vi "DDC (Four Channels).vi"(0 "data in":T1[](array[typedef]), 1 "reset":bool, 5 "start trigger":bool, 9 "enable":bool[](array[boolean]), 11 "ddc parameters":T2[](array[typedef]) {"frequency shift" format="%#.48g"}) -> (4 "data out":u32[](array[numeric]), 6 "number of overflows":u64[](array[numeric]), 10 "output valid":bool, 14 "dsp reset done":bool)   [LabVIEW 2016]
doc: "Digital downconverter (DDC). Implemented with FPGA-based DSP.\n\n<B>Input Parameters</B>\n\n<B>data in</B> is the I and Q data to be downconverted along with overflow information.\n\n<B>start trigger</B> triggers the Rx signal chain if an Rx stream is enabled.\n\n<B>enable</B> specifies which streams are enabled.\n\n<B>ddc parameters</B> are the downconversion parameters utilized by the DSP chain.\n\n<B>reset</B> the DSP downconversion signal chain.\n\n<B>Output Parameters</B>\n\n<B>dsp reset done</B> indicates that the DSP downconversion signal chain completed reset.\n\n<B>data out</B> is the downconverted data.\n\n<B>number of overflows</B> is the number of times the DSP chain overflowed on fixed point conversion of 'data in'.\n\n<B>output valid</B> specifies when 'data out' is valid."
uses:
  <instrlib>/_niInstr/DSP/v1/Shared/Public/IQ Data.ctl
  <instrlib>/_niInstr/DSP/v1/Shared/niInstr DSP v1 Shared.lvlib
  <instrlib>/_niInstr/DSP/v1/Shared/Public/IQ Impairments.ctl
  DDC Parameters.ctl
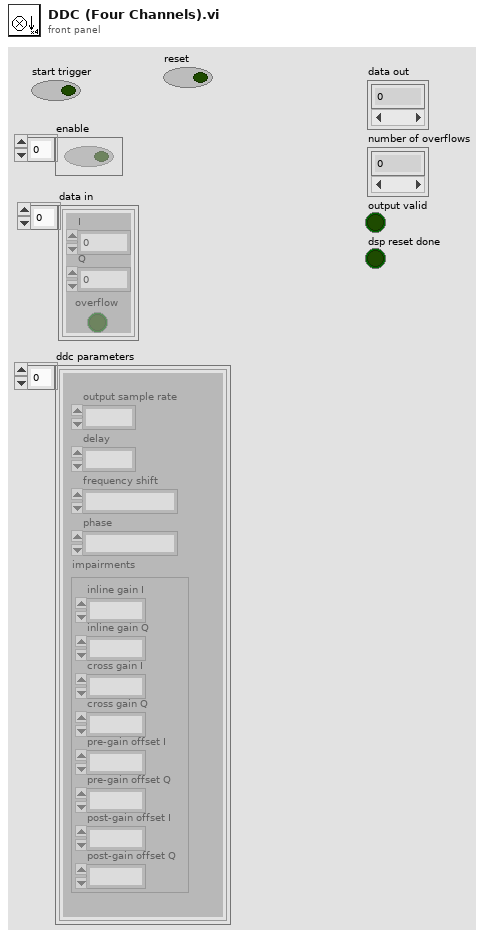
[diagram p1: front panel]
types:
  T1 = typedef "niInstr DSP v1 Shared.lvlib/IQ Data.ctl" = cluster{"I":fxp<+/-,18,1>, "Q":fxp<+/-,18,1>, "overflow":bool}
  T2 = typedef "DDC Parameters.ctl" = cluster{"output sample rate":fxp<+,48,1>, "delay":fxp<+/-,16,0>, "frequency shift":fxp<+/-,48,0>, "impairments":T3, "phase":fxp<+/-,21,0>}
  T3 = typedef "niInstr DSP v1 Shared.lvlib/IQ Impairments.ctl" = cluster{"inline gain I":fxp<+/-,18,1>, "inline gain Q":fxp<+/-,18,1>, "cross gain I":fxp<+/-,18,1>, "cross gain Q":fxp<+/-,18,1>, "pre-gain offset I":fxp<+/-,18,1>, "pre-gain offset Q":fxp<+/-,18,1>, "post-gain offset I":fxp<+/-,18,1>, "post-gain offset Q":fxp<+/-,18,1>}
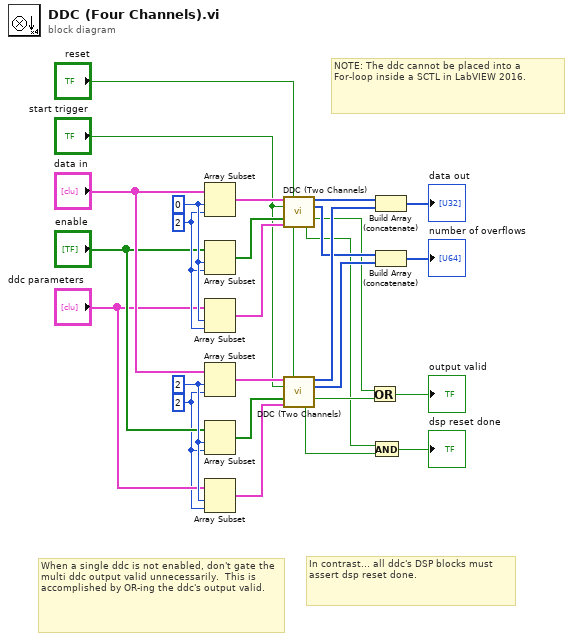
[diagram p0: block diagram]
diagram:
  w15 = 2 ("length")
  w20 = 2 ("index")
  w22 = 2 ("length")
  w23 = 0 ("index")
  # "NOTE: The ddc cannot be placed into a For-loop inside a SCTL in LabVIEW 2016."
  # "When a single ddc is not enabled, don't gate the multi ddc output valid unnecessarily.  This is accomplished by OR-ing the ddc's output valid."
  # "In contrast... all ddc's DSP blocks must assert dsp reset done."
  n1 = Array Subset(array="data in", index=w23, length=w22) -> (w25:T1[])
  n2 = Array Subset(array="enable", index=w23, length=w22) -> (w24:bool[])
  n3 = Array Subset(array="ddc parameters", index=w23, length=w22) -> (w21:T2[])
  n4 = Array Subset(array="data in", index=w20, length=w15) -> (w16:T1[])
  n5 = Array Subset(array="enable", index=w20, length=w15) -> (w13:bool[])
  n6 = Array Subset(array="ddc parameters", index=w20, length=w15) -> (w14:T2[])
  n7 = call "DDC (Two Channels).vi"("data in"=w25, "reset"="reset", "start trigger"="start trigger", "enable"=w24, "ddc parameters"=w21) -> ("data out"=w10:u32[], "number of overflows"=w6:u64[], "output valid"=w4:bool, "dsp reset done"=w1:bool)  [unwired: 7 in]
  n8 = call "DDC (Two Channels).vi"("data in"=w16, "reset"="reset", "start trigger"="start trigger", "enable"=w13, "ddc parameters"=w14) -> ("data out"=w9:u32[], "number of overflows"=w5:u64[], "output valid"=w3:bool, "dsp reset done"=w2:bool)  [unwired: 7 in]
  n9 = Or(x=w4, y=w3) -> (x .or. y?=→"output valid":bool)
  n10 = And(x=w1, y=w2) -> (x .and. y?=→"dsp reset done":bool)
  n11 = Build Array (concatenate)(w10, w9) -> (→"data out":u32[])
  n12 = Build Array (concatenate)(w6, w5) -> (→"number of overflows":u64[])
